vi "Factory (by name).vi"(0 "TTLDevice in":refnum<class "TTLControlledDevice.lvclass">, 7 "Class Name":string, 11 "error in (no error)":errorcluster) -> (4 "TTLDevice out":refnum<class "TTLControlledDevice.lvclass">, 15 "error out":errorcluster)   [LabVIEW 2020, in "TTLControlledDevice.lvclass"]
uses:
  TTLControlledDevice.lvclass
  TTLControlledDevice.lvclass/TTLControlledDevice.ctl
  WaterDelivery Class/TTLWaterDelivery.lvclass
  D:/Development/epl-tosca/LV Source/TTL VIs/Device Classes/Base Class/TTLControlledDevice.lvclass
  TCPControlledDevice/TCPControlledDevice.lvclass
  D:/Development/epl-vi-lib/Koop/KObject Class/KObject.lvclass
  D:/Development/epl-tosca/LV Source/TTL VIs/Device Classes/WaterDelivery Class/TTLWaterDelivery.lvclass
  D:/Development/epl-tosca/LV Source/TTL VIs/Device Classes/TCPControlledDevice/TCPControlledDevice.lvclass
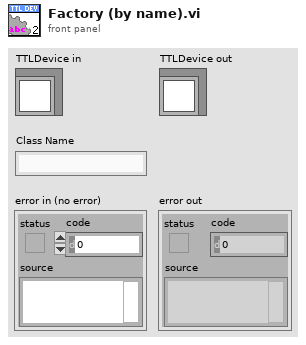
[diagram p1: front panel]
types:
  T1 = typedef "TTLControlledDevice.lvclass/Serialized.ctl" = cluster{"Name":string, "Line":string}
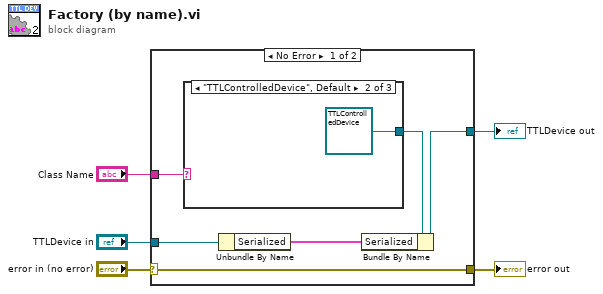
[diagram p0: block diagram]
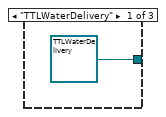
[diagram p2: hidden frame]
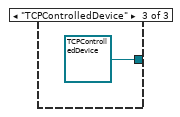
[diagram p3: hidden frame]
diagram:
  n1 = case shown="No Error" "error in (no error)" {
    selector: "error in (no error)" -> [w9 w16]
    tunnel: [w9 w16] -> w4
    tunnel: [w7 w15] -> w2
    tunnel: "TTLDevice in" -> [w8 w15]
    tunnel: "Class Name" -> [w10 _]
    frame No Error {
      n2 = case shown="\"TTLControlledDevice\", Default" w10 {
        tunnel: [refnum<class "TTLWaterDelivery.lvclass"> refnum ("TTLWater") refnum<class "TTLControlledDevice.lvclass"> refnum ("TTLDevice") refnum<class "TCPControlledDevice.lvclass"> refnum ("TCPControlledDevice")] -> w11
        frame "TTLWaterDelivery" {
        }
        frame "TTLControlledDevice", Default {
        }
        frame "TCPControlledDevice" {
        }
      }
      n3 = Unbundle By Name(w8) -> ("Serialized"=w6:T1)
      n4 = Bundle By Name(cluster=w11, "Serialized"=w6) -> (w7:refnum<class "TTLControlledDevice.lvclass">)
    }
    frame Error {
    }
  }
  "error out" <- w4
  "TTLDevice out" <- w2
